vi "ProcessModbusUpdatesSubnet3.vi"(11 "MockFAILC3Settings":T1={"ModbusTxDataFIFO"="MockbusPort2TxFIFO", "Code17Memory"="MockFAILC3Code17", "BufferUpdateFIFO"="MockFAILC3Command", "ModbusRxDataFIFO"="MockbusPort2RxFIFO", "Code18Memory"="MockFAILC3Code18", "Code65Memory"="MockFAILC3Code65", "Code66Memory"="MockFAILC3Code66", "Code67Memory"="MockFAILC3Code67", "Code72Memory"="MockFAILC3Code72", "Code80Memory"="MockFAILC3Code80", "Code110Memory"="MockFAILC3Code110", "CRCDataFIFO"="MockFAILC3CRCDataFIFO", "CRCCalculateFIFO"="MockFAILC3CRCCalculateFIFO", "CRCFIFO"="MockFAILC3CRCFIFO"}) -> ()   [LabVIEW 2016, in "FPGAMockFAILC.lvlib"]
uses:
  FPGAMockFAILC.lvlib
  FPGAMockHPILC/DataTypes/MockHPModbusUpdateLoopData.ctl
  FPGAMockHPILC/DataTypes/MockHPModbusUpdateStates.ctl
  <vilib>/Platform/TimedLoop/XDataNode/timing_clust.ctl
  <vilib>/Platform/TimedLoop/XDataNode/nitl_modes.ctl
  <vilib>/Platform/TimedLoop/XDataNode/wakeup.ctl
  <vilib>/rvi/Emulation/niFpgaSctlEmulationGetInTimedLoop.vi
  <vilib>/rvi/Emulation/niFpgaEmulationReportErrorSimple.vi
  <vilib>/rvi/Emulation/niFpgaGetClockAttributes.vi
  <vilib>/rvi/Emulation/niFpgaCriticalErrorInLSC.vi
  <vilib>/rvi/DataTransferAndStorage/Container/Common/niFpgaContainerExecOnDevCompGetState.vi
  <vilib>/rvi/Emulation/niFpgaEmulationIsFPGAContextNoSignature.vi
  <vilib>/rvi/errors/niFpgaSetErrorForExecOnDevCompSimple.vi
  <vilib>/rvi/eio/common/nirviEmuReportErrorAndStop.vi
  <vilib>/rvi/DataTransferAndStorage/Container/Common/niFpgaContainerGetUniqueNameForEmu.vi
  <vilib>/rvi/FIFO/Fifo_Resource/nirvififoEmulationSetSize.vi
  <vilib>/rvi/FIFO/Fifo_Resource/nirviFifoEmulationQueueMgr.vi
  <instcachedir>/0/nirviFifoEmulationQueueMgr_E5CAEC123FF24DC58D834DCA3CDAA9B5.lvgen/nirviFifoEmulationQueueMgr_E5CAEC123FF24DC58D834DCA3CDAA9B5_002.vi
  <vilib>/rvi/FIFO/Fifo_Resource/nirvififoEmulationDetermineInputValidOut.vi
  <vilib>/rvi/FIFO/Fifo_Resource/nirvififoEmulationCreateLock.vi
  <vilib>/rvi/Emulation/niFpgaProcessEmulError.vi
  <vilib>/rvi/FIFO/Fifo_Resource/nirvififoEmulationObtainLock.vi
  <vilib>/rvi/FIFO/Fifo_Resource/nirvififoEmulationReleaseLock.vi
  <vilib>/rvi/occurrence/nirviWaitOnOccurrenceBase.vi
  <vilib>/rvi/errors/nirviReportUnexpectedCaseInternalError.vi
  <vilib>/rvi/errors/nirviReportUnexpectedCaseInternalError (U32).vi
  <vilib>/Utility/error.llb/Clear Errors.vi
  <vilib>/rvi/interface/RandomDataEmulation/niFpgaRandomDataHandleErrors.vi
  <instcachedir>/0/nirviFifoEmulationQueueMgr_E5CAEC123FF24DC58D834DCA3CDAA9B5.lvgen/nirviFifoEmulationQueueMgr_E5CAEC123FF24DC58D834DCA3CDAA9B5_000.vi
  <vilib>/rvi/Memory/Memory_Emulation/niFpgaMemoryEmulationCacheClearOnFirstRun.vi
  <vilib>/rvi/Memory/Memory_Emulation/nirvimemoryEmulationManagerCache_MakeExclusive.vi
  <vilib>/rvi/Memory/Memory_Emulation/niFpgaMemoryEmulationValidateCache.vi
  <vilib>/rvi/Memory/Memory_Emulation/nirvimemoryEmulationManagerCache_InsertValue.vi
  <vilib>/rvi/Memory/Memory_Emulation/nirvimemoryEmulationManagerCache_ReleaseExclusive.vi
  <vilib>/rvi/Memory/Memory_Emulation/nirvimemoryEmulationManagerCache_GetValue.vi
  <vilib>/rvi/Memory/Memory_Emulation/nirvimemoryEmulationManagerCache_SetValue.vi
  <vilib>/rvi/Emulation/niFpgaSctlEmulationResourceMgr.vi
  <instcachedir>/0/nirviFifoEmulationQueueMgr_E5CAEC123FF24DC58D834DCA3CDAA9B5.lvgen/nirviFifoEmulationQueueMgr_E5CAEC123FF24DC58D834DCA3CDAA9B5_001.vi
  <vilib>/Platform/TimedLoop/XDataNode/XDataNode.xnode
  <vilib>/rvi/DataTransferAndStorage/Container/XNode/niFpgaContainer.xnode
  <vilib>/rvi/FIFO/Fifo_Resource/niFpgaFifoEmulationRefIn.vi
  <vilib>/rvi/Memory/Memory_Emulation/niFpgaMemoryEmulationRefIn.vi
  FPGAMockHPILC/FPGAMockHPILC.lvlib
  <vilib>/Platform/TimedLoop/XDataNode/XDNodeRunTimeDep.lvlib
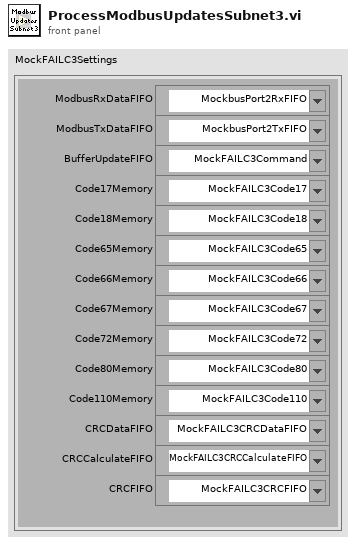
[diagram p1: front panel]
types:
  T1 = cluster{"ModbusTxDataFIFO":refnum<k21>, "Code17Memory":refnum<k21>, "BufferUpdateFIFO":refnum<k21>, "ModbusRxDataFIFO":refnum<k21>, "Code18Memory":refnum<k21>, "Code65Memory":refnum<k21>, "Code66Memory":refnum<k21>, "Code67Memory":refnum<k21>, "Code72Memory":refnum<k21>, "Code80Memory":refnum<k21>, "Code110Memory":refnum<k21>, "CRCDataFIFO":refnum<k21>, "CRCCalculateFIFO":refnum<k21>, "CRCFIFO":refnum<k21>}
  T2 = typedef "FPGAMockHPILC.lvlib/MockHPModbusUpdateLoopData.ctl" = cluster{"ModbusUpdateLoopStates":T3, "Address":u8, "Function":u8, "ResponseLength":u8, "ResponseIndex":u8, "Index":u8, "Data":u16, "DelayTicks":u32}
  T3 = typedef "FPGAMockHPILC.lvlib/MockHPModbusUpdateStates.ctl" = enum16{"ReadModbusPort", "ProcessModbusData", "DelayMicroseconds", "WriteAddress", "WriteFunction", "WriteData", "WriteCRCLSB", "WriteCRCMSB", "WriteEndOfFrame", "CalculateCRC"}
  T4 = typedef "XDNodeRunTimeDep.lvlib/timing_clust.ctl" = cluster{"Expected End [f-1]":u64, "Actual End [f-1]":u64, "Finished Late? [f-1]":bool, "Expected End [i-1]":u64, "Actual End [i-1]":u64, "Finished Late? [i-1]":bool, "Expected Start [i]":u64, "Actual Start [i]":u64, "Expected Start [f]":u64, "Actual Start [f]":u64, "Source Name":string, "Structure Name":string, "Period":i64, "Deadline":i64, "Offset":i64, "Start":i64, "Priority":i32, "Timeout":i32, "Mode":T5, "Wakeup Reason":T6, "Error":errorcluster, "Source Type":string, "Secondary Source Type":string, "Global End Time":u64, "Global Start Time":u64, "Frame Duration":u64, "Iteration Duration":u64, "Assigned CPU":i32, "I/O Scan Engine Mode":u32}
  T5 = typedef "XDNodeRunTimeDep.lvlib/nitl_modes.ctl" = enum32{"No Change", "Process missed periods, maintain original phase", "Discard missed periods, maintain original phase", "Process missed periods, ignore original phase", "Discard missed periods, ignore original phase"}
  T6 = typedef "XDNodeRunTimeDep.lvlib/wakeup.ctl" = enum32{"Normal", "Aborted", "Asynchronous wakeup", "Timing source error", "Timed loop error", "Timeout"}
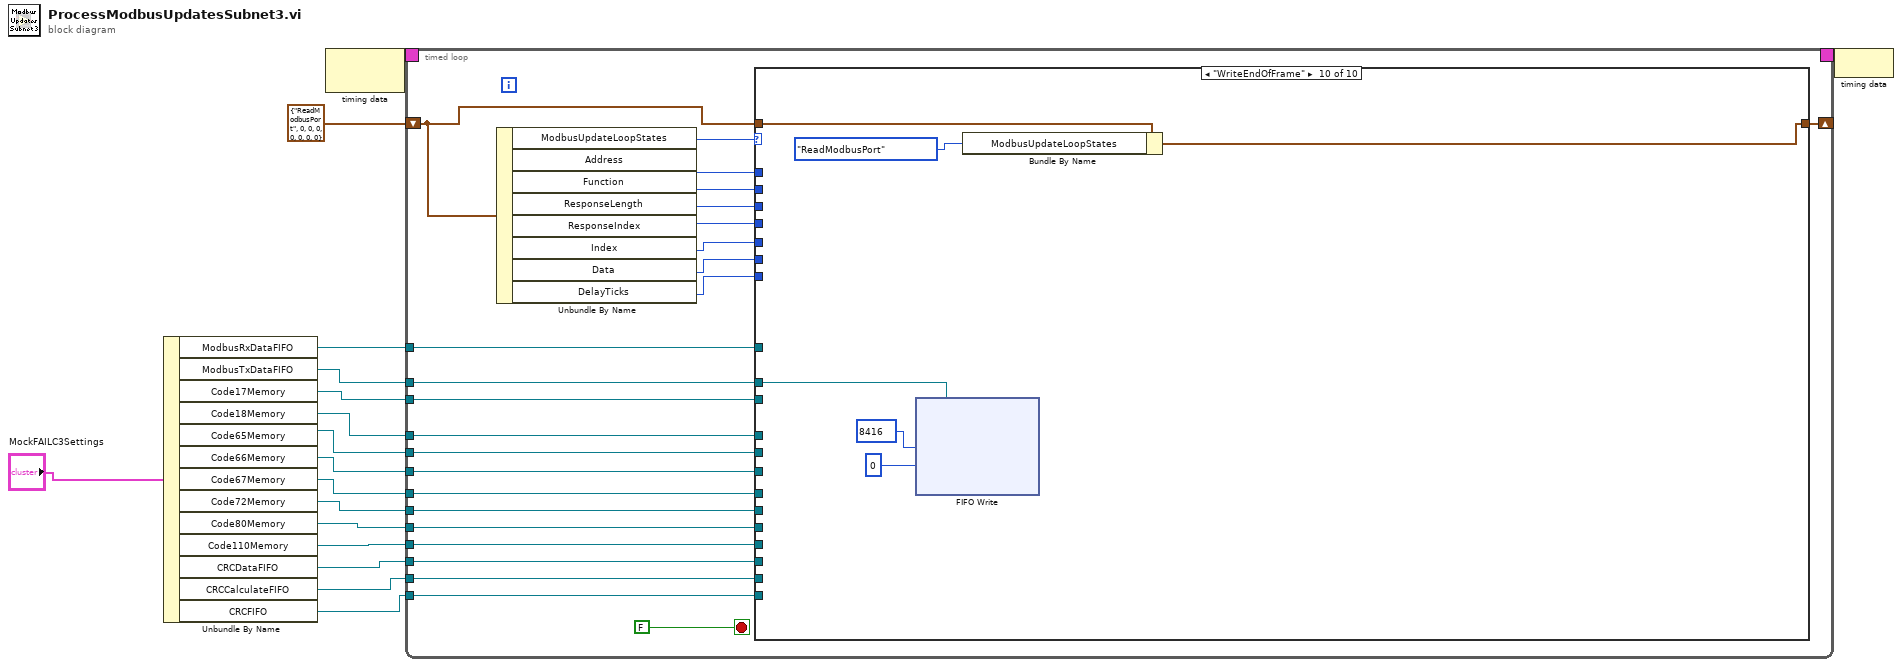
[diagram p0: block diagram]
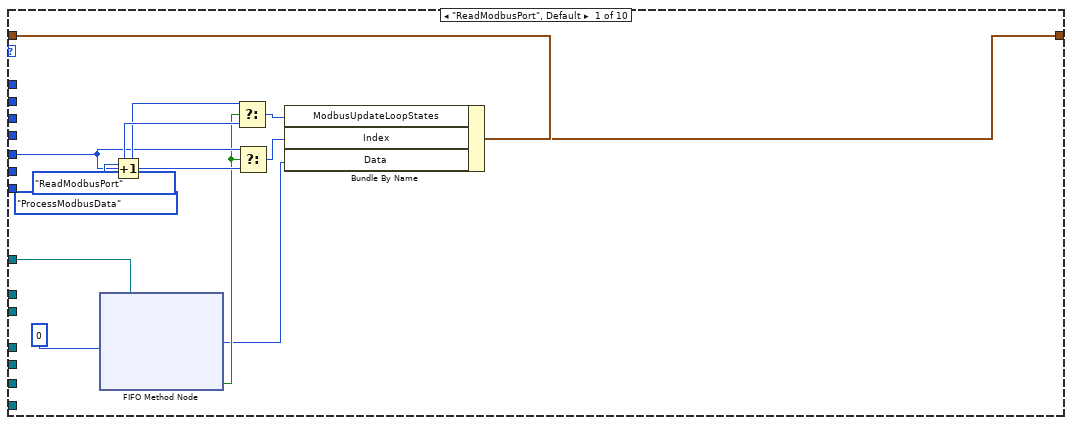
[diagram p2: hidden frame]
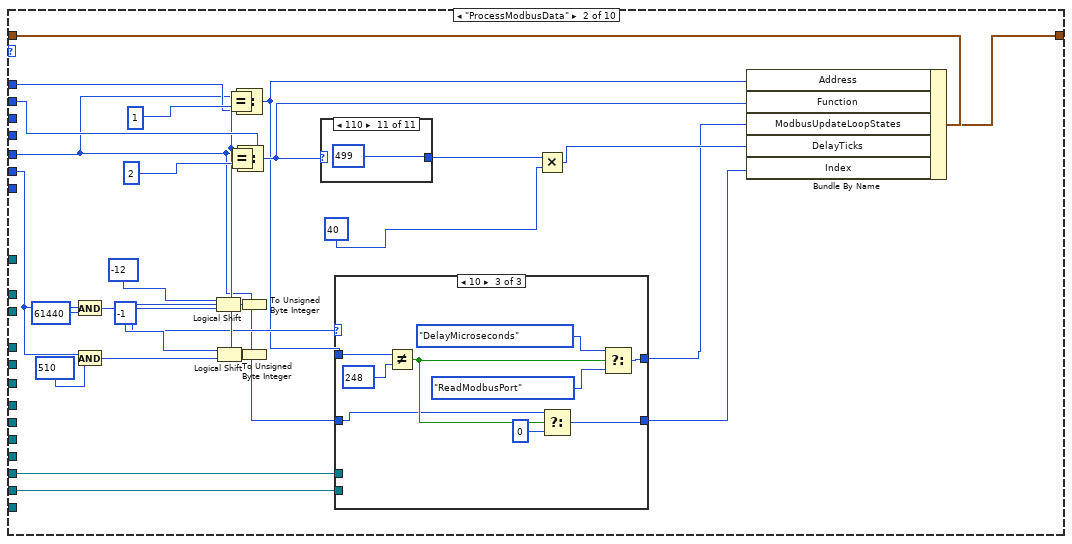
[diagram p3: hidden frame]
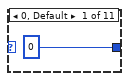
[diagram p4: hidden frame]
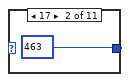
[diagram p5: hidden frame]
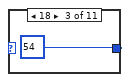
[diagram p6: hidden frame]
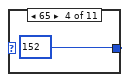
[diagram p7: hidden frame]
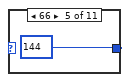
[diagram p8: hidden frame]
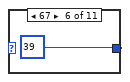
[diagram p9: hidden frame]
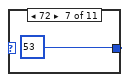
[diagram p10: hidden frame]
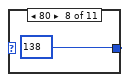
[diagram p11: hidden frame]
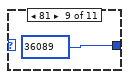
[diagram p12: hidden frame]
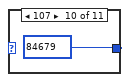
[diagram p13: hidden frame]
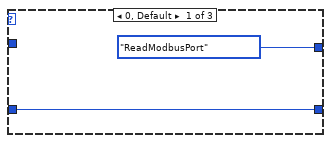
[diagram p14: hidden frame]
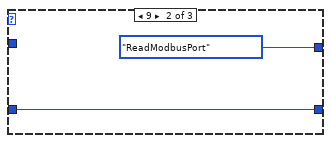
[diagram p15: hidden frame]
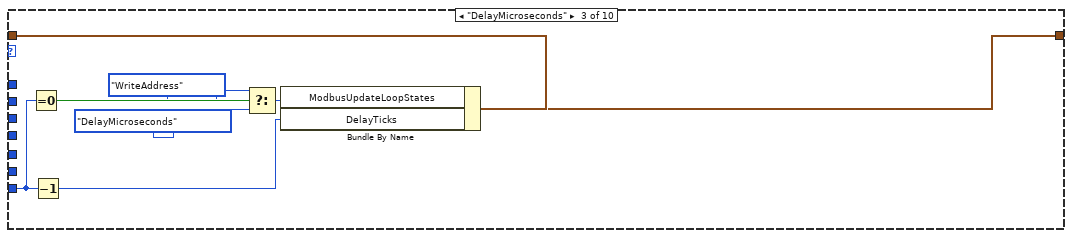
[diagram p16: hidden frame]
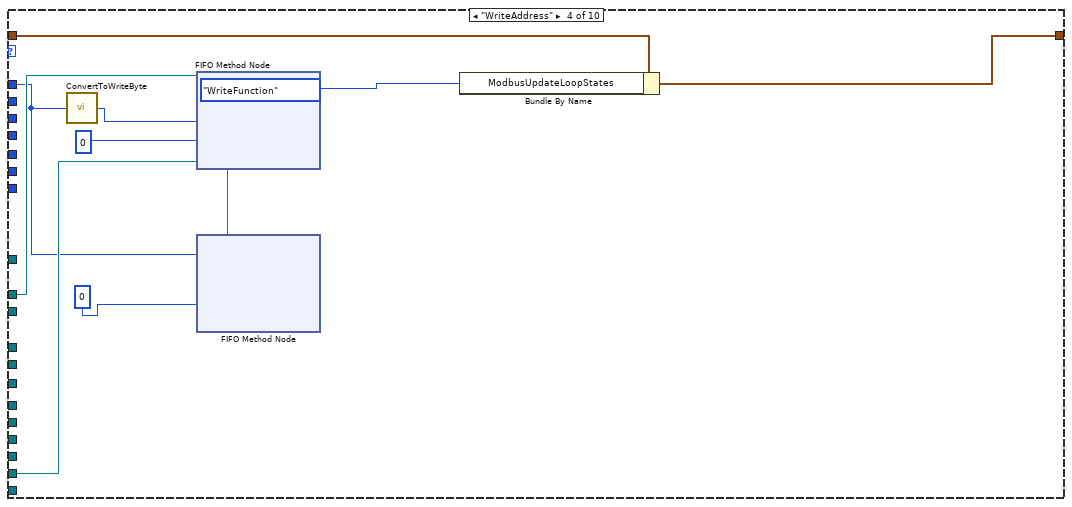
[diagram p17: hidden frame]
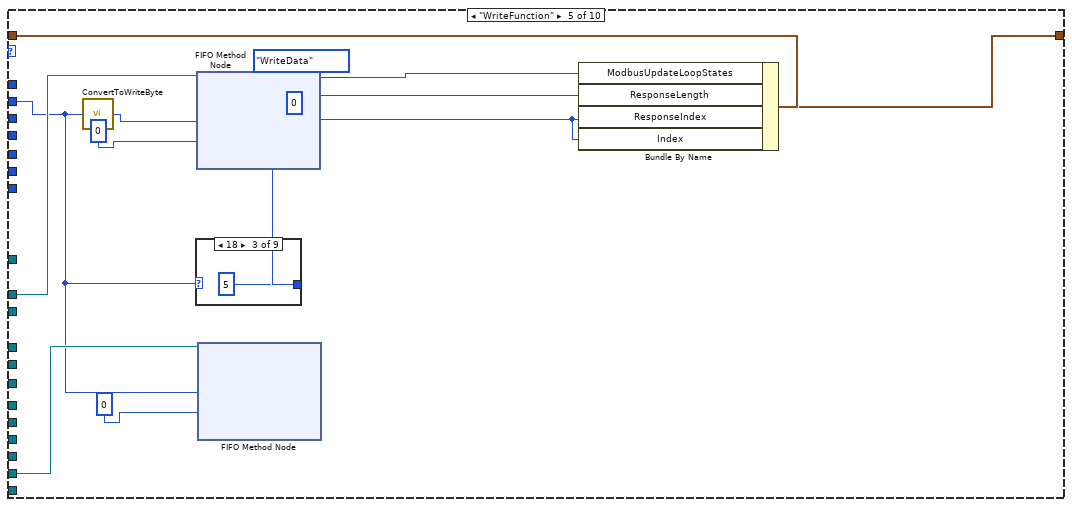
[diagram p18: hidden frame]
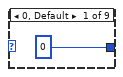
[diagram p19: hidden frame]
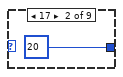
[diagram p20: hidden frame]
diagram:
  n1 = Unbundle By Name("MockFAILC3Settings") -> ("ModbusRxDataFIFO"=w14:refnum<k21>, "ModbusTxDataFIFO"=w13:refnum<k21>, "Code17Memory"=w12:refnum<k21>, "Code18Memory"=w11:refnum<k21>, "Code65Memory"=w10:refnum<k21>, "Code66Memory"=w9:refnum<k21>, "Code67Memory"=w8:refnum<k21>, "Code72Memory"=w7:refnum<k21>, "Code80Memory"=w6:refnum<k21>, "Code110Memory"=w5:refnum<k21>, "CRCDataFIFO"=w4:refnum<k21>, "CRCCalculateFIFO"=w3:refnum<k21>, "CRCFIFO"=w2:refnum<k21>)
  n2 = node-c288() -> (w17:T4)  [unwired: 1 in]
  n3 = timed-loop {
    shift-right: [w36] -> _
    shift-left: T2 {"ModbusUpdateLoopStates"=enum."ReadModbusPort", "Address"=0, "Function"=0, "ResponseLength"=0, "ResponseIndex"=0, "Index"=0, "Data"=0, "DelayTicks"=0} ("MockHPBufferUpdateLoopData") -> [w35]
    timing: w17 -> [_]
    timing-out: [_] -> w16
    tunnel: w14 -> [w34]
    tunnel: w13 -> [w30]
    tunnel: w12 -> [w29]
    tunnel: w11 -> [w28]
    tunnel: w10 -> [w27]
    tunnel: w9 -> [w26]
    tunnel: w8 -> [w25]
    tunnel: w7 -> [w24]
    tunnel: w6 -> [w23]
    tunnel: w5 -> [w22]
    tunnel: w4 -> [w18]
    tunnel: w3 -> [w21]
    tunnel: w2 -> [w20]
    stop <- FALSE stop-if-true
    n4 = Unbundle By Name(w35) -> ("ModbusUpdateLoopStates"=w41:T3, "Address"=w40:u8, "Function"=w39:u8, "ResponseLength"=w38:u8, "ResponseIndex"=w37:u8, "Index"=w33:u8, "Data"=w32:u16, "DelayTicks"=w19:u32)
    n5 = case shown="\"WriteEndOfFrame\"" w41 {
      tunnel: w40 -> [_ w58 _ w116 _ w168 _ _ _ _]
      tunnel: w39 -> [_ w67 _ _ w125 w171 _ _ _ _]
      tunnel: w38 -> [_ _ _ _ _ w148 _ _ _ _]
      tunnel: w37 -> [_ _ _ _ _ w145 _ _ _ _]
      tunnel: [w44 w81 w113 w118 w129 w172 w232 w243 w257 w266] -> w36
      tunnel: w35 -> [w45 w82 w114 w120 w131 w173 w236 w244 w258 w270]
      tunnel: w34 -> [w53 _ _ _ _ _ _ _ _ _]
      tunnel: w33 -> [w48 w55 _ _ _ _ _ _ _ _]
      tunnel: w32 -> [_ w74 _ _ _ _ _ _ _ _]
      tunnel: w30 -> [_ _ _ w123 w134 w164 _ w238 w252 w269]
      tunnel: w29 -> [_ _ _ _ _ w170 _ _ _ _]
      tunnel: w28 -> [_ _ _ _ _ w163 _ _ _ _]
      tunnel: w27 -> [_ _ _ _ _ w162 _ _ _ _]
      tunnel: w26 -> [_ _ _ _ _ w161 _ _ _ _]
      tunnel: w25 -> [_ _ _ _ _ w160 _ _ _ _]
      tunnel: w24 -> [_ _ _ _ _ w159 _ _ _ _]
      tunnel: w23 -> [_ _ _ _ _ w158 _ _ _ _]
      tunnel: w22 -> [_ _ _ _ _ w157 _ _ _ _]
      tunnel: w18 -> [_ w71 _ w117 w126 w146 _ _ _ _]
      tunnel: w21 -> [_ w70 _ _ _ _ w235 _ _ _]
      tunnel: w20 -> [_ _ _ _ _ _ _ w242 w256 _]
      tunnel: w19 -> [_ _ w108 _ _ _ _ _ _ _]
      frame "ReadModbusPort", Default {
        n6 = xnode ("FIFO Method Node")("Timeout"=0, "FIFO In"=w53) -> ("Element"=w42:u16, "Timed Out?"=w43:bool)  [unwired: 1 out]
        n7 = Increment(x=w48) -> (x+1=w49:u8)
        n8 = Select(t=MockHPModbusUpdateStates."ReadModbusPort", s=w43, f=MockHPModbusUpdateStates."ProcessModbusData") -> (s? t:f=w47:T3)
        n9 = Select(t=w48, s=w43, f=w49) -> (s? t:f=w46:u8)
        n10 = Bundle By Name(cluster=w45, "ModbusUpdateLoopStates"=w47, "Index"=w46, "Data"=w42) -> (w44:T2)
      }
      frame "ProcessModbusData" {
        n11 = And(x=w74, y=u16 61440) -> (x .and. y?=w76:u16)
        n12 = And(x=w74, y=u16 510) -> (x .and. y?=w79:u16)
        n13 = Logical Shift(y=i16 -12, x=w76) -> (x << y=w64:u16)
        n14 = Logical Shift(y=i16 -1, x=w79) -> (x << y=w66:u16)
        n15 = Equal?(x=w55, y=u8 1) -> (x = y?=w72:bool)
        n16 = Equal?(x=w55, y=u8 2) -> (x = y?=w69:bool)
        n17 = To Unsigned Byte Integer(number=w64) -> (unsigned 8bit integer=w63:u8)
        n18 = To Unsigned Byte Integer(number=w66) -> (unsigned 8bit integer=w65:u8)
        n19 = Select(t=w65, s=w72, f=w58) -> (s? t:f=w57:u8)
        n20 = Select(t=w65, s=w69, f=w67) -> (s? t:f=w62:u8)
        n21 = case shown="110" w62 {
          tunnel: [u32 0 ("Count(uSec)") u32 463 ("Count(uSec)") u32 54 ("Count(uSec)") u32 152 ("Count(uSec)") u32 144 ("Count(uSec)") u32 39 ("Count(uSec)") u32 53 ("Count(uSec)") u32 138 ("Count(uSec)") u32 36089 ("Count(uSec)") u32 84679 ("Count(uSec)") u32 499 ("Count(uSec)")] -> w61
          frame 0, Default {
          }
          frame 17 {
          }
          frame 18 {
          }
          frame 65 {
          }
          frame 66 {
          }
          frame 67 {
          }
          frame 72 {
          }
          frame 80 {
          }
          frame 81 {
          }
          frame 107 {
          }
          frame 110 {
          }
        }
        n22 = case shown="10" w63 {
          tunnel: w71 -> [_ _ _]
          tunnel: w70 -> [_ _ _]
          tunnel: [MockHPModbusUpdateStates."ReadModbusPort" ("f") MockHPModbusUpdateStates."ReadModbusPort" ("f") w106] -> w56
          tunnel: w57 -> [_ _ w102]
          tunnel: w55 -> [w94 w96 w100]
          tunnel: [w94 w96 w98] -> w54
          frame 0, Default {
          }
          frame 9 {
          }
          frame 10 {
            n23 = Not Equal?(x=w102, y=u8 248) -> (x != y?=w101:bool)
            n24 = Select(t=w100, s=w101, f=u8 0) -> (s? t:f=w98:u8)
            n25 = Select(t=MockHPModbusUpdateStates."DelayMicroseconds" ("f"), s=w101, f=MockHPModbusUpdateStates."ReadModbusPort") -> (s? t:f=w106:T3)
          }
        }
        n26 = Multiply(x=w61, y=u32 40) -> (x*y=w59:u32)
        n27 = Bundle By Name(cluster=w82, "Address"=w57, "Function"=w62, "ModbusUpdateLoopStates"=w56, "DelayTicks"=w59, "Index"=w54) -> (w81:T2)
      }
      frame "DelayMicroseconds" {
        n28 = Equal To 0?(x=w108) -> (x = 0?=w112:bool)
        n29 = Decrement(x=w108) -> (x-1=w107:u32)
        n30 = Select(t=MockHPModbusUpdateStates."WriteAddress", s=w112, f=MockHPModbusUpdateStates."DelayMicroseconds") -> (s? t:f=w111:T3)
        n31 = Bundle By Name(cluster=w114, "ModbusUpdateLoopStates"=w111, "DelayTicks"=w107) -> (w113:T2)
      }
      frame "WriteAddress" {
        n32 = call "ConvertToWriteByte.vi"("Input"=w116) -> ("Output"=w122:u16)
        n33 = xnode ("FIFO Method Node")("Element"=w122, "Timeout"=0, "FIFO In"=w123) -> ()  [unwired: 2 out]
        n34 = xnode ("FIFO Method Node")("Element"=w116, "Timeout"=0, "FIFO In"=w117) -> ()  [unwired: 2 out]
        n35 = Bundle By Name(cluster=w120, "ModbusUpdateLoopStates"=MockHPModbusUpdateStates."WriteFunction") -> (w118:T2)
      }
      frame "WriteFunction" {
        w127 = u8 0 ("ResponseIndex")
        n36 = call "ConvertToWriteByte.vi"("Input"=w125) -> ("Output"=w133:u16)
        n37 = case shown="18" w125 {
          tunnel: [u8 0 ("ResponseLength") u8 20 ("ResponseLength") u8 5 ("ResponseLength") u8 2 ("ResponseLength") u8 9 ("ResponseLength") u8 9 ("ResponseLength") u8 1 ("ResponseLength") u8 1 ("ResponseLength") u8 96 ("ResponseLength")] -> w128
          frame 0, Default {
          }
          frame 17 {
          }
          frame 18 {
          }
          frame 65 {
          }
          frame 66 {
          }
          frame 67 {
          }
          frame 72 {
          }
          frame 80 {
          }
          frame 110 {
          }
        }
        n38 = xnode ("FIFO Method Node")("Element"=w133, "Timeout"=0, "FIFO In"=w134) -> ()  [unwired: 2 out]
        n39 = xnode ("FIFO Method Node")("Element"=w125, "Timeout"=0, "FIFO In"=w126) -> ()  [unwired: 2 out]
        n40 = Bundle By Name(cluster=w131, "ModbusUpdateLoopStates"=MockHPModbusUpdateStates."WriteData", "ResponseLength"=w128, "ResponseIndex"=w127, "Index"=w127) -> (w129:T2)
      }
      frame "WriteData" {
        n41 = Decrement(x=w168) -> (x-1=w169:u8)
        n42 = Multiply(x=w169, y=w148) -> (x*y=w167:u8)
        n43 = Add(x=w167, y=w145) -> (x+y=w166:u8)
        n44 = case shown="110" w171 {
          tunnel: w170 -> [_ w184 _ _ _ _ _ _ _]
          tunnel: w166 -> [_ w188 w194 w200 w206 w212 w218 w224 w230]
          tunnel: [u8 0 ("Data") w185 w191 w197 w203 w209 w215 w221 w227] -> w165
          tunnel: [FALSE TRUE TRUE TRUE TRUE TRUE TRUE TRUE TRUE] -> w150
          tunnel: w163 -> [_ _ w190 _ _ _ _ _ _]
          tunnel: w162 -> [_ _ _ w196 _ _ _ _ _]
          tunnel: w161 -> [_ _ _ _ w202 _ _ _ _]
          tunnel: w160 -> [_ _ _ _ _ w208 _ _ _]
          tunnel: w159 -> [_ _ _ _ _ _ w214 _ _]
          tunnel: w158 -> [_ _ _ _ _ _ _ w220 _]
          tunnel: w157 -> [_ _ _ _ _ _ _ _ w226]
          tunnel: [TRUE FALSE ("t") FALSE FALSE FALSE FALSE FALSE FALSE FALSE] -> w144
          frame 0, Default {
          }
          frame 17 {
            n45 = xnode ("Memory Method Node")("Address"=w188, "Memory In"=w184) -> ("Data"=w186:u8)  [unwired: 1 out]
            n46 = feedback-in #1(w186) -> ()
            n47 = feedback #1() -> (w185:u8)  [unwired: 1 in]
          }
          frame 18 {
            n48 = xnode ("Memory Method Node")("Address"=w194, "Memory In"=w190) -> ("Data"=w192:u8)  [unwired: 1 out]
            n49 = feedback-in #2(w192) -> ()
            n50 = feedback #2() -> (w191:u8)  [unwired: 1 in]
          }
          frame 65 {
            n51 = xnode ("Memory Method Node")("Address"=w200, "Memory In"=w196) -> ("Data"=w198:u8)  [unwired: 1 out]
            n52 = feedback-in #3(w198) -> ()
            n53 = feedback #3() -> (w197:u8)  [unwired: 1 in]
          }
          frame 66 {
            n54 = xnode ("Memory Method Node")("Address"=w206, "Memory In"=w202) -> ("Data"=w204:u8)  [unwired: 1 out]
            n55 = feedback-in #4(w204) -> ()
            n56 = feedback #4() -> (w203:u8)  [unwired: 1 in]
          }
          frame 67 {
            n57 = xnode ("Memory Method Node")("Address"=w212, "Memory In"=w208) -> ("Data"=w210:u8)  [unwired: 1 out]
            n58 = feedback-in #5(w210) -> ()
            n59 = feedback #5() -> (w209:u8)  [unwired: 1 in]
          }
          frame 72 {
            n60 = xnode ("Memory Method Node")("Address"=w218, "Memory In"=w214) -> ("Data"=w216:u8)  [unwired: 1 out]
            n61 = feedback-in #6(w216) -> ()
            n62 = feedback #6() -> (w215:u8)  [unwired: 1 in]
          }
          frame 80 {
            n63 = xnode ("Memory Method Node")("Address"=w224, "Memory In"=w220) -> ("Data"=w222:u8)  [unwired: 1 out]
            n64 = feedback-in #7(w222) -> ()
            n65 = feedback #7() -> (w221:u8)  [unwired: 1 in]
          }
          frame 110 {
            n66 = xnode ("Memory Method Node")("Address"=w230, "Memory In"=w226) -> ("Data"=w228:u8)  [unwired: 1 out]
            n67 = feedback-in #8(w228) -> ()
            n68 = feedback #8() -> (w227:u8)  [unwired: 1 in]
          }
        }
        n69 = Increment(x=w145) -> (x+1=w152:u8)
        n70 = Increment(x=w148) -> (x+1=w147:u8)
        n71 = Equal To 0?(x=w145) -> (x = 0?=w151:bool)
        n72 = Equal?(x=w147, y=w152) -> (x = y?=w156:bool)
        n73 = Select(t=w144, s=w151, f=w150) -> (s? t:f=w149:bool)
        n74 = case shown="True" w149 {
          tunnel: w165 -> [_ w175]
          tunnel: w164 -> [_ w177]
          tunnel: w146 -> [_ w176]
          frame False {
          }
          frame True {
            n75 = call "ConvertToWriteByte.vi"("Input"=w175) -> ("Output"=w178:u16)
            n76 = xnode ("FIFO Method Node")("Element"=w178, "Timeout"=0, "FIFO In"=w177) -> ()  [unwired: 2 out]
            n77 = xnode ("FIFO Method Node")("Element"=w175, "Timeout"=0, "FIFO In"=w176) -> ()  [unwired: 2 out]
          }
        }
        n78 = Select(t=MockHPModbusUpdateStates."CalculateCRC", s=w156, f=MockHPModbusUpdateStates."WriteData") -> (s? t:f=w153:T3)
        n79 = Bundle By Name(cluster=w173, "ModbusUpdateLoopStates"=w153, "ResponseIndex"=w152) -> (w172:T2)
      }
      frame "CalculateCRC" {
        n80 = xnode ("FIFO Write")("Element"=TRUE, "Timeout"=0, "FIFO In"=w235) -> ()  [unwired: 2 out]
        n81 = Bundle By Name(cluster=w236, "ModbusUpdateLoopStates"=MockHPModbusUpdateStates."WriteCRCLSB") -> (w232:T2)
      }
      frame "WriteCRCLSB" {
        n82 = xnode ("FIFO Read")("Timeout"=0, "FIFO In"=w242) -> ("Element"=w239:u8, "Timed Out?"=w240:bool)  [unwired: 1 out]
        n83 = case shown="False" w240 {
          tunnel: w239 -> [w249 _]
          tunnel: w238 -> [w248 _]
          tunnel: [MockHPModbusUpdateStates."WriteCRCMSB" ("ModbusUpdateLoopStates") MockHPModbusUpdateStates."WriteCRCLSB" ("ModbusUpdateLoopStates")] -> w237
          frame False {
            n84 = call "ConvertToWriteByte.vi"("Input"=w249) -> ("Output"=w247:u16)
            n85 = xnode ("FIFO Write")("Element"=w247, "Timeout"=0, "FIFO In"=w248) -> ()  [unwired: 2 out]
          }
          frame True {
          }
        }
        n86 = Bundle By Name(cluster=w244, "ModbusUpdateLoopStates"=w237) -> (w243:T2)
      }
      frame "WriteCRCMSB" {
        n87 = xnode ("FIFO Read")("Timeout"=0, "FIFO In"=w256) -> ("Element"=w253:u8, "Timed Out?"=w254:bool)  [unwired: 1 out]
        n88 = case shown="True" w254 {
          tunnel: w253 -> [w263 _]
          tunnel: w252 -> [w262 _]
          tunnel: [MockHPModbusUpdateStates."WriteEndOfFrame" ("ModbusUpdateLoopStates") MockHPModbusUpdateStates."WriteCRCMSB" ("ModbusUpdateLoopStates")] -> w251
          frame False {
            n89 = call "ConvertToWriteByte.vi"("Input"=w263) -> ("Output"=w261:u16)
            n90 = xnode ("FIFO Write")("Element"=w261, "Timeout"=0, "FIFO In"=w262) -> ()  [unwired: 2 out]
          }
          frame True {
          }
        }
        n91 = Bundle By Name(cluster=w258, "ModbusUpdateLoopStates"=w251) -> (w257:T2)
      }
      frame "WriteEndOfFrame" {
        n92 = xnode ("FIFO Write")("Element"=u16 8416, "Timeout"=0, "FIFO In"=w269) -> ()  [unwired: 2 out]
        n93 = Bundle By Name(cluster=w270, "ModbusUpdateLoopStates"=MockHPModbusUpdateStates."ReadModbusPort") -> (w266:T2)
      }
    }
  }
  n94 = node-c288(w16) -> ()
